vi "Stream Configuration.vi"() -> ()   [LabVIEW 2016, in "Lab Streaming Layer.lvlib"]
uses:
  Lab Streaming Layer.lvlib
  Custom Controls/lsl_channel_format.ctl
panel:
  out "xml":string
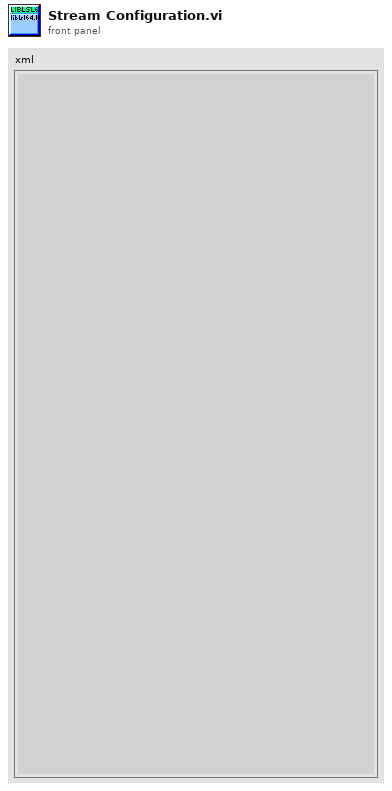
[diagram p1: front panel]
types:
  T1 = typedef "liblsl-LabVIEW.lvlib/lsl_channel_format.ctl" = u32
  T2 = typedef "liblsl-LabVIEW.lvlib/lsl_streaminfo.ctl" = u64
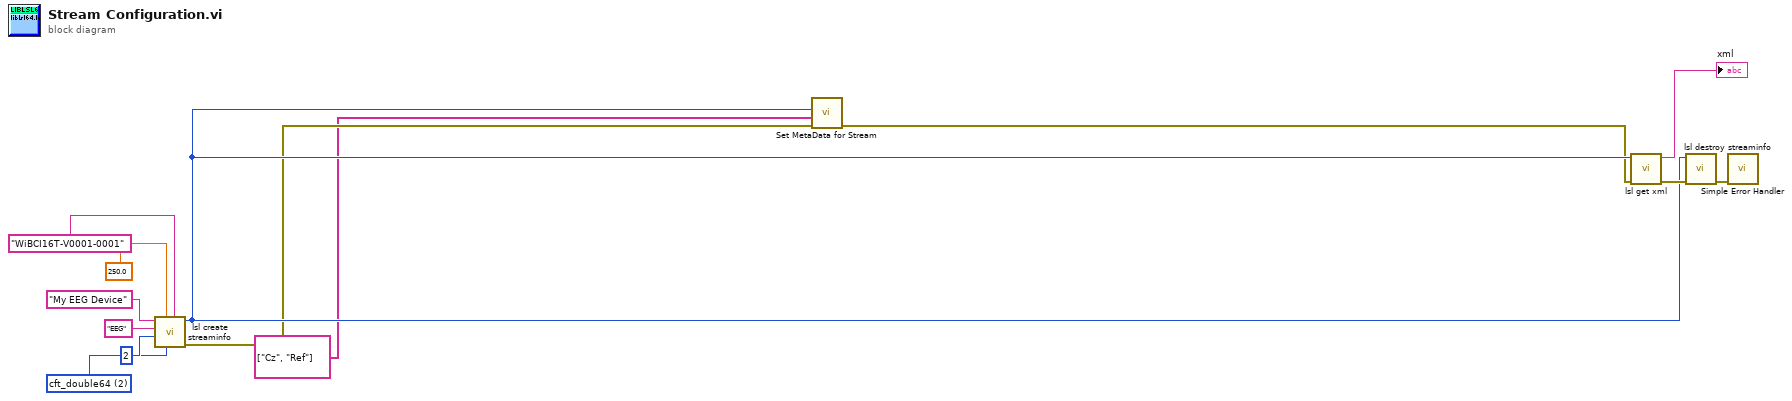
[diagram p0: block diagram]
diagram:
  w8 = T1 2 items=["cft_float32"=1, "cft_double64"=2, "cft_string"=3, "cft_int32"=4, "cft_int16"=5, "cft_int8"=6, "cft_int64"=7, "cft_undefined"=0] ("channel_format")
  n1 = call "lsl create streaminfo.vi"("source_id"="WiBCI16T-V0001-0001", "channel_format"=w8, "samplingrate"=250.0, "channel_count"=2, "type"="EEG", "name"="My EEG Device") -> ("error out"=w4:errorcluster, "streaminfo"=w5:T2)  [unwired: 4 in]
  n2 = call "Set MetaData for Stream.vi"("error in"=w4, "Ch Names"=string[] ["Cz", "Ref"], "streaminfo"=w5) -> ("error out"=w1:errorcluster)  [unwired: 8 in]
  n3 = call "lsl get xml.vi"("error in (no error)"=w1, "streaminfo"=w5) -> ("error out"=w6:errorcluster, "xml"=→"xml":string)  [unwired: 8 in]
  n4 = call "lsl destroy streaminfo.vi"("error in (no error)"=w6, "streaminfo"=w5) -> ("error out"=w7:errorcluster)  [unwired: 9 in]
  n5 = call <vilib>:"Simple Error Handler.vi"("error in (no error)"=w7) -> ()  [unwired: 4 in, 5 out]
